vi "Zero_Instruments.vi"(3 "Mode":T5, 5 "Traverse line In":T2 {"Carrier_2 Q (l/min)" format="%#.2f"; "Row Duration (mins)" format="%#.1f"; "Row No" min=0; "Trace Gas Concentration (%)" min=0.0 format="%#_4f"; "Carrier_1 Q (l/min)" format="%#.2f"; "Tunnel Speed" format="%#.2f"; "Start X" format="%#.2f"; "Start Y" format="%#.2f"; "Start Z" format="%#.2f"; "End X" format="%#.2f"; "End Y" format="%#.2f"; "End Z" format="%#.2f"; "Averaging time (min)" min=0.0 format="%#.2f"}) -> (0 "Error Message":string, 1 "Status":T1, 2 "Traverse line Out":T2 {"Carrier_2 Q (l/min)" format="%#.2f"; "Row Duration (mins)" format="%#.1f"; "Row No" min=0; "Trace Gas Concentration (%)" min=0.0 format="%#_4f"; "Carrier_1 Q (l/min)" format="%#.2f"; "Tunnel Speed" format="%#.2f"; "Start X" format="%#.2f"; "Start Y" format="%#.2f"; "Start Z" format="%#.2f"; "End X" format="%#.2f"; "End Y" format="%#.2f"; "End Z" format="%#.2f"; "Averaging time (min)" min=0.0 format="%#.2f"})   [LabVIEW 2017]
uses:
  Gen Trav/Traverse_cluster.ctl
  Gen Trav/Spacing.ctl
  Controls/Multi_run_mode.ctl
  Controls/User_Specific_mode.ctl
  Gen Trav/Multi_Run_Status.ctl
  Controls/Setup.ctl
  Controls/Save_Data.ctl
  Camera Server/Camera enum/Camera resolution.ctl
  Globals/Meas_global.vi
  <vilib>/Analysis/NI_AALPro.lvlib
  <vilib>/Analysis/NI_AALBase.lvlib
panel:
  # "X           Y            Z"
  # "Start"
  # "End"
  # "X           Y            Z"
  # "Start"
  # "End"
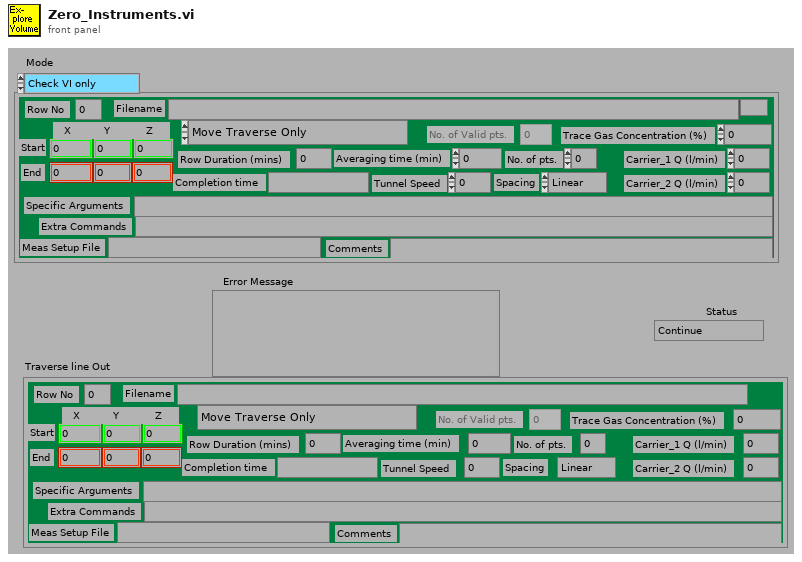
[diagram p1: front panel]
types:
  T1 = typedef "Multi_Run_Status.ctl" = enum16{"Continue", "Continue with Error", "Jump to Next Point", "Jump to Next Row", "Jump To Fall Back", "Terminate Run"}
  T2 = typedef "Traverse_cluster.ctl" = cluster{"Start X":sgl, "Start Y":sgl, "Start Z":sgl, "End X":sgl, "End Y":sgl, "End Z":sgl, "No. of pts.":i32, "Spacing":T3, "Filename":path, "Tunnel Speed":dbl, "Averaging time (min)":dbl, "Extra Commands":string, "Carrier_1 Q (l/min)":dbl, "Carrier_2 Q (l/min)":dbl, "Trace Gas Concentration (%)":dbl, "Specific Arguments":string, "Comments":string, "Row No":i32, "Row Type Selector":T4, "Completion time":string, "Row Duration (mins)":dbl, "No. of Valid pts.":i32, "Meas Setup File":string}
  T3 = typedef "Spacing.ctl" = enum16{"Linear", "Log", "Gauss", "Specified", "N/A"}
  T4 = typedef "Multi_run_mode.ctl" = enum16{"Move Traverse Only", "Set Tunnel Speed Only", "Set Source Only", "Set Measurement Conditions", "Single Measurement", "Vertical Profile", "Lateral Profile", "Longitudinal Profile", "Explore Volume", "Multi-Axis Profile", "Auto Calibrate", "Meas Fast FID Bkgnd", "Check Beam Power", "Scanning Valve Measurement", "Run VI Named:", "Set ADAM Ch", "Wait (minutes)", "Send Message", "Synchronize With:", "Fall Back to this Row", "Turn Off Row Repeating", "Blank Row", "Traverse 3D Volume"}
  T5 = typedef "User_Specific_mode.ctl" = enum16{"Check VI only", "Run VI"}
  T6 = typedef "Save_Data.ctl" = enum16{"Save No Data", "Save Data"}
  T7 = typedef "Setup.ctl" = enum16{"Run Program", "Show Setup", "Save Current Setup", "Setup Front Panel"}
  T8 = typedef "Analysis_info_cluster.ctl" = cluster{"Colour":u32, "Inst type":T9, "Inst name":string, "Symbol":string, "Code name":string, "Extra Info":string, "Inst Array":T10, "Extra Titles":string[], "Extra Values":string[], "U":dbl, "u^2":dbl, "u^3":dbl, "u^4":dbl, "Skew_u":dbl, "Kurt_u":dbl, "Sd Error in Mean":dbl, "% u'/U":dbl, "X":dbl, "Y":dbl, "Z":dbl, "Timescale integral Estimate":dbl, "Sd Error in Variance":dbl, "Calib File":path, "Calib Constants":dbl[], "Output Position":bool, "Full Stats":bool, "Av Sampling Rate":dbl, "Av No of Samples":dbl, "Total Meas Time (s)":dbl, "ADAM Ch Name":string, "Max value":dbl, "Min value":dbl, "Sync Delay Time (s)":dbl}
  T9 = typedef "Inst_type.ctl" = enum16{"Propeller anemometer", "Raw voltage", "Pressure Transducer", "Pitot-static tube", "Preston tube", "Hot wire", "Cross wire 1", "Cross wire 2", "Generic Linear", "Generic Polynomial", "Generic BackPoly", "Fast FID", "Thermocouple", "Cold wire", "Pulsed Wire", "LDA Vel", "LDA Tran time", "LDA Arr time", "Microphone"}
  T10 = typedef "Instrument_Array.ctl" = enum16{"PWA", "LDA", "Analogue"}
  T11 = typedef "Time_Trace_Cluster.ctl" = cluster{"Weighting":dbl[], "Time (s)":dbl[], "Voltage":dbl[], "Eng Values":dbl[]}
  T12 = typedef "Camera resolution.ctl" = u8
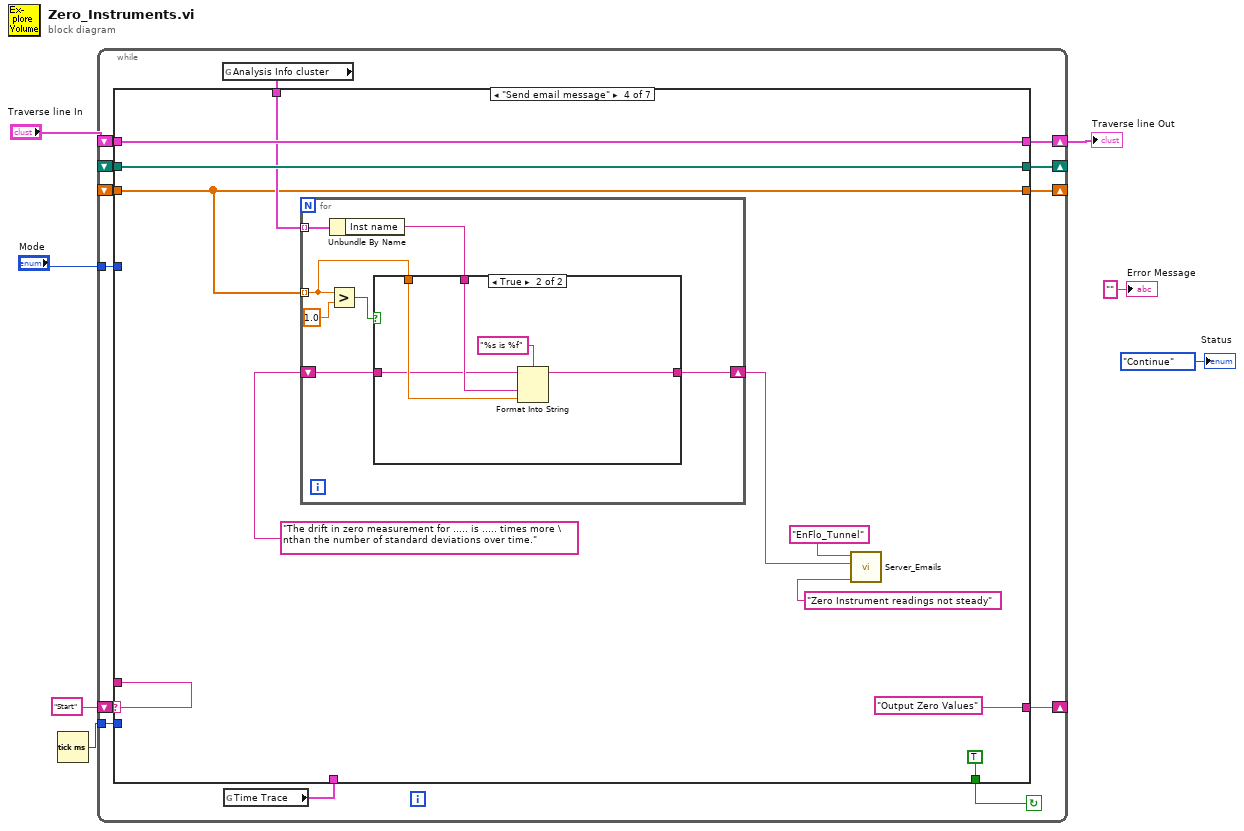
[diagram p0: block diagram]
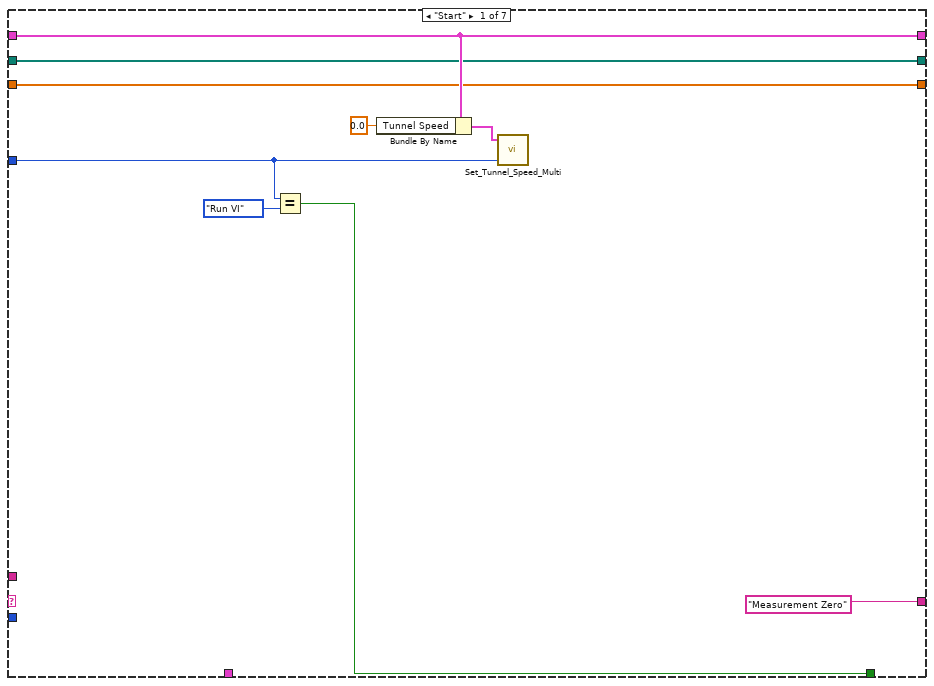
[diagram p2: hidden frame]
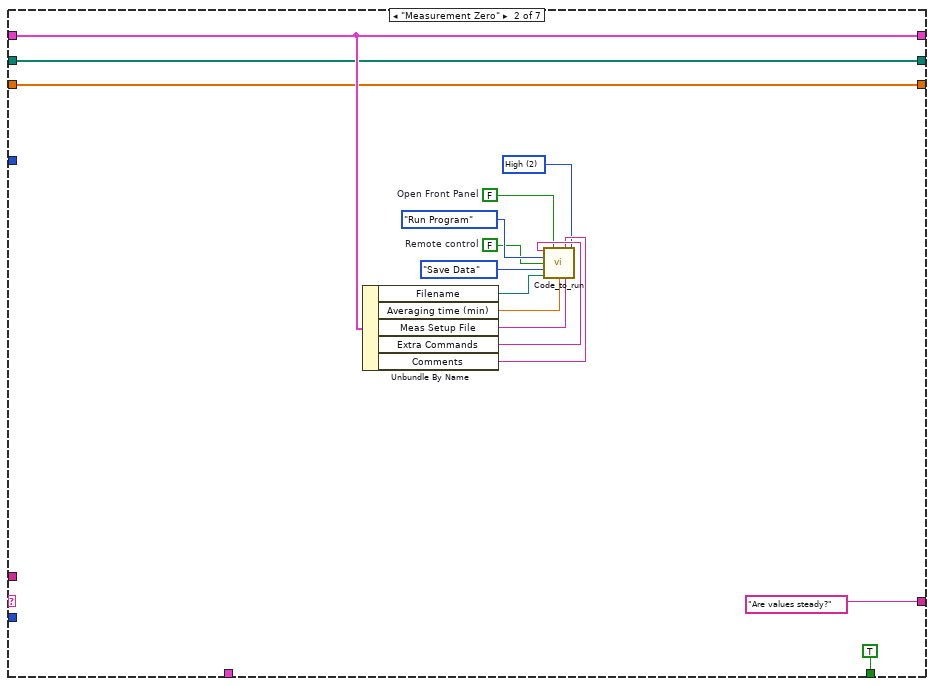
[diagram p3: hidden frame]
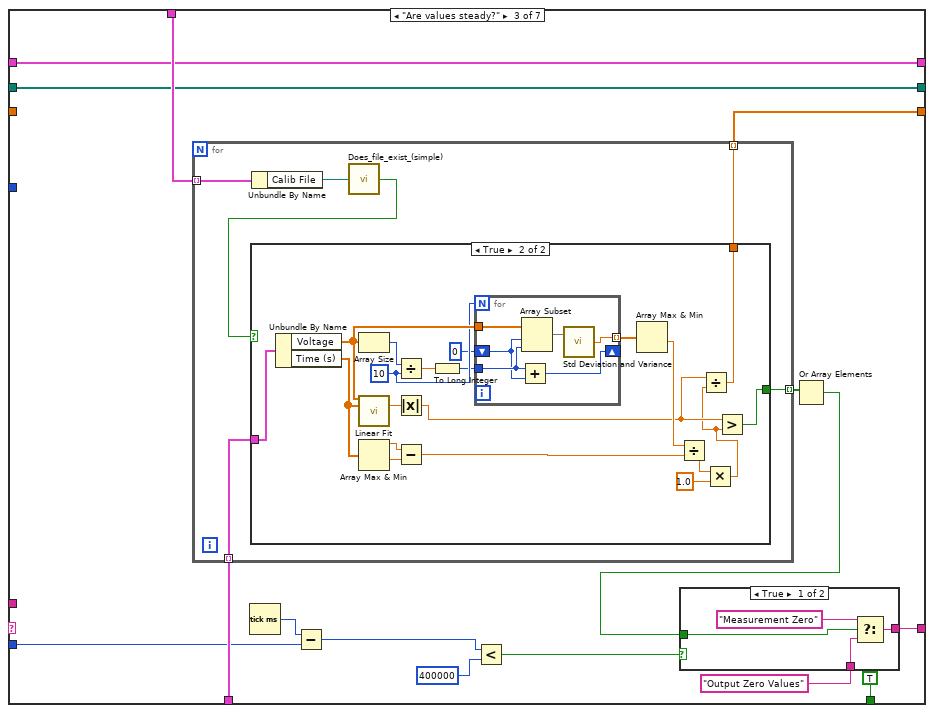
[diagram p4: hidden frame]
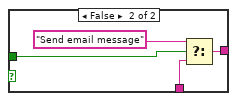
[diagram p5: hidden frame]
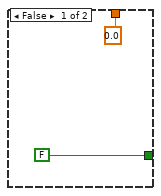
[diagram p6: hidden frame]
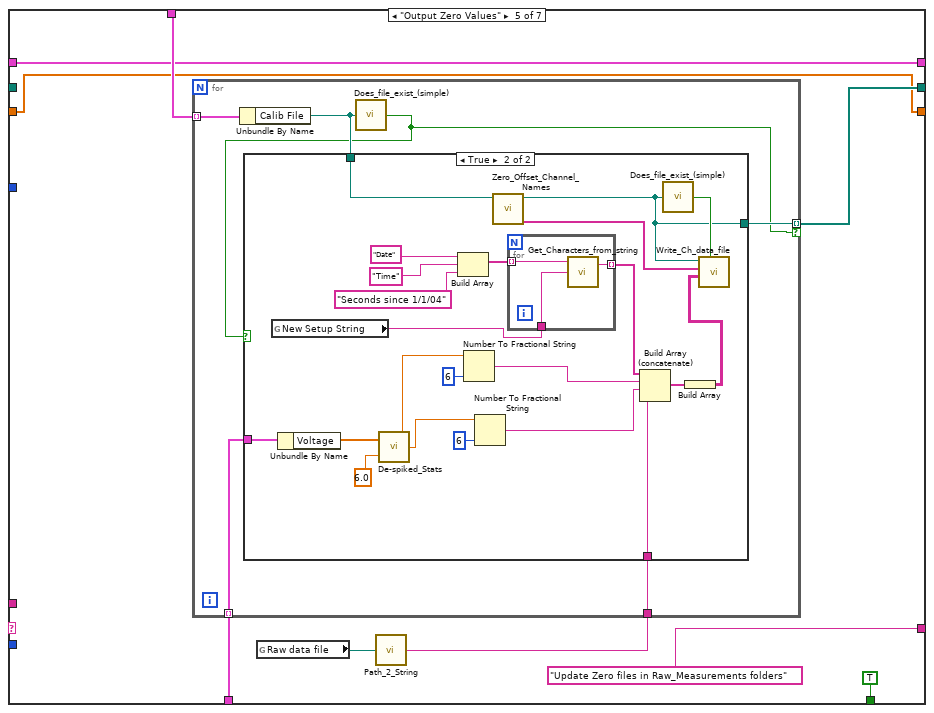
[diagram p8: hidden frame]
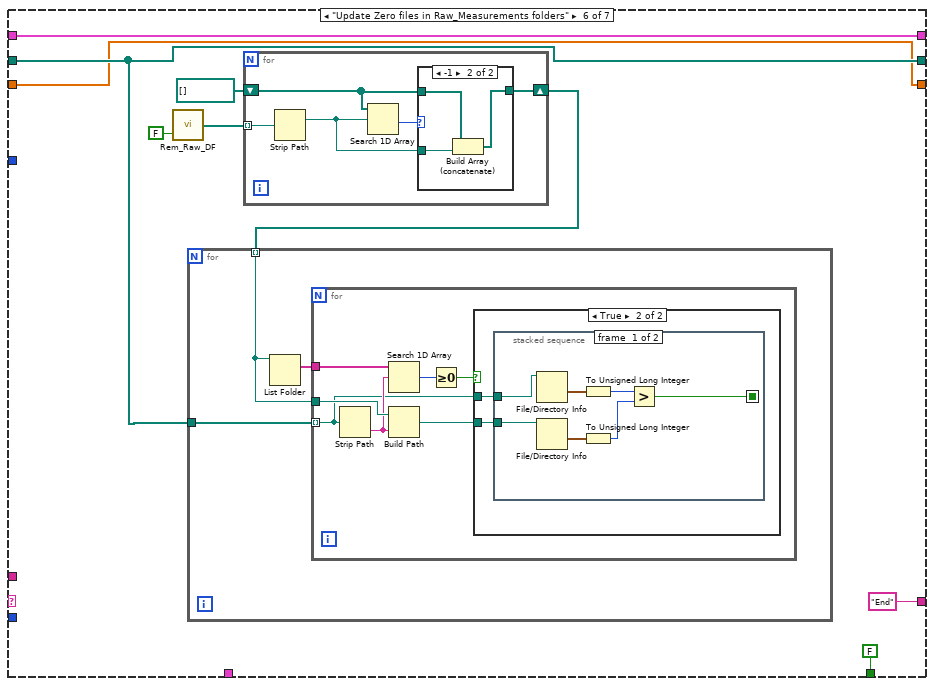
[diagram p10: hidden frame]
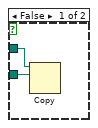
[diagram p11: hidden frame]
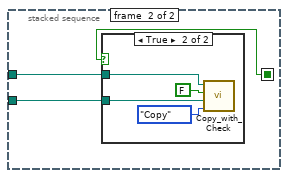
[diagram p12: hidden frame]
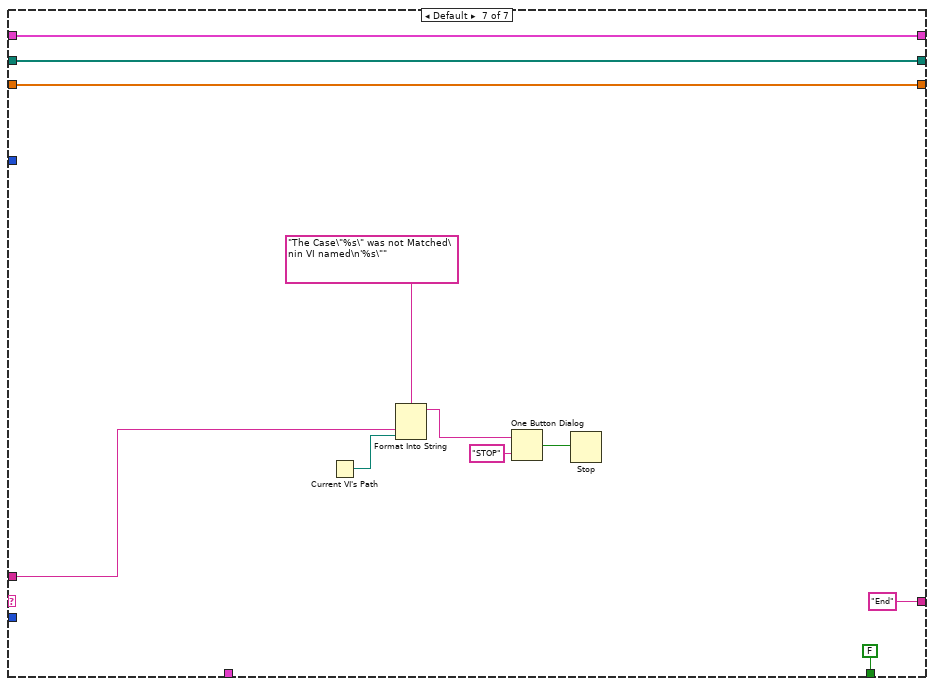
[diagram p15: hidden frame]
diagram:
  n1 = Tick Count (ms)() -> (millisecond timer value=w1:u32)
  n2 = while {
    shift-right: [w16] -> _
    shift-left: "Start" -> [w15]
    shift-right: [w17] -> w5
    shift-left: "Traverse line In" -> [w19]
    tunnel: "Mode" -> [w18]
    tunnel: w1 -> [w12]
    shift-right: [w11] -> _
    shift-left: _ -> [w10]
    shift-right: [w9] -> _
    shift-left: _ -> [w8]
    stop <- w20 continue-if-true
    n3 = global read "Meas_global.vi" "Analysis Info cluster"() -> (w13:T8[])
    n4 = global read "Meas_global.vi" "Time Trace"() -> (w14:T11[])
    n5 = case shown="\"Send email message\"" w15 {
      tunnel: [w24 TRUE TRUE TRUE TRUE FALSE FALSE] -> w20
      tunnel: w19 -> [w27 w33 w56 w110 w130 w174 w214]
      tunnel: w18 -> [w26 _ _ _ _ _ _]
      tunnel: [w27 w33 w56 w110 w130 w174 w214] -> w17
      tunnel: ["Measurement Zero" "Are values steady?" w53 "Output Zero Values" "Update Zero files in Raw_Measurements folders" "End" "End"] -> w16
      tunnel: w15 -> [_ _ _ _ _ _ w217]
      tunnel: w14 -> [_ _ w58 _ w132 _ _]
      tunnel: w13 -> [_ _ w57 w108 w131 _ _]
      tunnel: w12 -> [_ _ w51 _ _ _ _]
      tunnel: [w22 w31 w49 w109 w126 w169 w213] -> w11
      tunnel: w10 -> [w22 w31 w49 w109 _ w169 w213]
      tunnel: [w21 w30 w45 w102 w125 w166 w212] -> w9
      tunnel: w8 -> [w21 w30 _ w102 w125 w166 w212]
      frame "Start" {
        n6 = Equal?(x=w26, y=User_Specific_mode."Run VI") -> (x = y?=w24:bool)
        n7 = Bundle By Name(cluster=w27, "Tunnel Speed"=0.0) -> (w29:T2)
        n8 = call "Set_Tunnel_Speed_Multi.vi"("Simulate/Run"=w26, "Traverse line"=w29) -> ()  [unwired: 4 out]
      }
      frame "Measurement Zero" {
        w37 = T12 2 items=["Low", "Med.", "High", "Max."] ("Camera Resolution")
        w38 = FALSE  # Open Front Panel
        w35 = FALSE  # Remote control
        n9 = Unbundle By Name(w33) -> ("Filename"=w43:path, "Averaging time (min)"=w42:dbl, "Meas Setup File"=w41:string, "Extra Commands"=w40:string, "Comments"=w39:string)
        n10 = call "Code_to_run.vi"("Extra command String"=w40, "Open Front Panel"=w38, "Current Row Comments"=w39, "Camera Resolution"=w37, "setup"=Setup."Run Program", "Remote control"=w35, "File"=Save_Data."Save Data", "Results Filename"=w43, "Averaging time (min)"=w42, "Setup filename"=w41) -> ()  [unwired: 2 in, 4 out]
      }
      frame "Are values steady?" {
        n11 = for {
          tunnel: w57 -> [w73] mode=indexing
          tunnel: w58 -> [w70] mode=indexing
          tunnel: [w69] -> w55 mode=indexing
          tunnel: [w68] -> w45 mode=indexing
          n12 = Unbundle By Name(w73) -> ("Calib File"=w72:path)
          n13 = call "Does_file_exist_(simple).vi"("Pathname"=w72) -> ("exists?"=w71:bool)
          n14 = case shown="True" w71 {
            tunnel: w70 -> [_ w82]
            tunnel: [FALSE w80] -> w69
            tunnel: [0.0 w76] -> w68
            frame False {
            }
            frame True {
              w88 = 10 ("y")
              n15 = Unbundle By Name(w82) -> ("Voltage"=w95:dbl[], "Time (s)"=w90:dbl[])
              n16 = Array Size(array=w95) -> (size(s)=w84:i32)
              n17 = call <vilib>:"Linear Fit.vi"("Y"=w95, "X"=w90) -> ("slope"=w83:dbl)  [unwired: 9 in, 4 out]
              n18 = Array Max & Min(array=w90) -> (max value=w91:dbl, min value=w92:dbl)  [unwired: 2 out]
              n19 = Divide(x=w84, y=w88) -> (x/y=w86:dbl)
              n20 = Absolute Value(x=w83) -> (abs(x)=w78:dbl)
              n21 = Subtract(x=w91, y=w92) -> (x-y=w94:dbl)
              n22 = To Long Integer(number=w86) -> (32bit integer=w87:i32)
              n23 = for {
                N: w88 -> [_]
                tunnel: w95 -> [w101]
                shift-right: [w98] -> _
                shift-left: 0 ("y") -> [w99]
                tunnel: w87 -> [w100]
                tunnel: [w96] -> w89 mode=indexing
                n24 = Add(x=w100, y=w99) -> (x+y=w98:i32)
                n25 = Array Subset(array=w101, index=w99, length=w100) -> (w97:dbl[])
                n26 = call <vilib>:"Std Deviation and Variance.vi"("X"=w97) -> ("standard deviation"=w96:dbl)  [unwired: 1 in, 2 out]
              }
              n27 = Array Max & Min(array=w89) -> (min value=w93:dbl)  [unwired: 3 out]
              n28 = Divide(x=w93, y=w94) -> (x/y=w81:dbl)
              n29 = Multiply(x=w81, y=1.0) -> (x*y=w77:dbl)
              n30 = Divide(x=w78, y=w77) -> (x/y=w76:dbl)
              n31 = Greater?(x=w78, y=w77) -> (0:w80:bool)
            }
          }
        }
        n32 = Tick Count (ms)() -> (millisecond timer value=w52:u32)
        n33 = Subtract(x=w52, y=w51) -> (x-y=w50:u32)
        n34 = Less?(x=w50, y=u32 400000) -> (x < y?=w48:bool)
        n35 = Or Array Elements(Boolean array=w55) -> (logical OR=w47:bool)
        n36 = case shown="True" w48 {
          tunnel: [w63 w67] -> w53
          tunnel: w47 -> [w61 w66]
          tunnel: "Output Zero Values" -> [w60 w64]
          frame True {
            n37 = Select(t="Measurement Zero", s=w61, f=w60) -> (s? t:f=w63:string)
          }
          frame False {
            n38 = Select(t="Send email message", s=w66, f=w64) -> (s? t:f=w67:string)
          }
        }
      }
      frame "Send email message" {
        n39 = for {
          tunnel: w108 -> [w118] mode=indexing
          tunnel: w102 -> [w114] mode=indexing
          shift-right: [w112] -> w103
          shift-left: "The drift in zero measurement for ..... is ..... times more \nthan the number of standard deviations over time." -> [w113]
          n40 = Greater?(x=w114, y=1.0) -> (0:w116:bool)
          n41 = Unbundle By Name(w118) -> ("Inst name"=w115:string)
          n42 = case shown="True" w116 {
            tunnel: w115 -> [_ w124]
            tunnel: w114 -> [_ w123]
            tunnel: w113 -> [w119 w122]
            tunnel: [w119 w121] -> w112
            frame False {
            }
            frame True {
              n43 = Format Into String(format string="%s is %f", initial string=w122, w124, w123) -> (resulting string=w121:string)  [unwired: 1 in, 1 out]
            }
          }
        }
        n44 = call "Server_Emails.vi"("Client Name Contains"="EnFlo_Tunnel", "Message"=w103, "Subject"="Zero Instrument readings not steady" ("Error Type")) -> ()  [unwired: 2 in, 3 out]
      }
      frame "Output Zero Values" {
        n45 = global read "Meas_global.vi" "Raw data file"() -> (w128:path)
        n46 = call "Path_2_String.vi"("Real Path"=w128) -> ("Path String"=w127:string)
        n47 = for {
          tunnel: w131 -> [w139] mode=indexing
          tunnel: w132 -> [w138] mode=indexing
          tunnel: w127 -> [w137]
          tunnel: [w135] -> w126 mode=indexing if=w134
          n48 = Unbundle By Name(w139) -> ("Calib File"=w136:path)
          n49 = call "Does_file_exist_(simple).vi"("Pathname"=w136) -> ("exists?"=w134:bool)
          n50 = case shown="True" w134 {
            tunnel: w138 -> [_ w162]
            tunnel: w137 -> [_ w146]
            tunnel: w136 -> [w140 w142]
            tunnel: [w140 w141] -> w135
            frame False {
            }
            frame True {
              n51 = global read "Meas_global.vi" "New Setup String"() -> (w150:string)
              n52 = Unbundle By Name(w162) -> ("Voltage"=w160:dbl[])
              n53 = call "De-spiked_Stats.vi"("Raw Signal"=w160, "No of st dev to chop at"=6.0) -> ("mean"=w156:dbl, "standard deviation"=w157:dbl)  [unwired: 1 out]
              n54 = Build Array("Date", "Time", "Seconds since 1/1/04") -> (w151:string[])
              n55 = Number To Fractional String(number=w156, precision (6)=i16 6) -> (F-format string=w148:string)  [unwired: 2 out]
              n56 = Number To Fractional String(number=w157, precision (6)=i16 6) -> (F-format string=w147:string)  [unwired: 2 out]
              n57 = call "Zero_Offset_Channel_Names.vi"("Calib Filename"=w142) -> ("Channel names"=w145:string[], "Zero Filename"=w141:path)  [unwired: 3 in, 2 out]
              n58 = for {
                tunnel: w151 -> [w165] mode=indexing
                tunnel: w150 -> [w164]
                tunnel: [w163] -> w149 mode=indexing
                n59 = call "Get_Characters_from_string.vi"("Input string"=w164, "Variable name"=w165) -> ("Value"=w163:string)  [unwired: 1 in, 1 out]
              }
              n60 = Build Array (concatenate)(w149, w148, w147, w146) -> (w144:string[])
              n61 = call "Does_file_exist_(simple).vi"("Pathname"=w141) -> ("exists?"=w155:bool)
              n62 = Build Array(w144) -> (w143:string[][])
              n63 = call "Write_Ch_data_file.vi"("exists?"=w155, "Channel Values"=w143, "Channel names"=w145, "Filename"=w141) -> ()  [unwired: 4 in, 4 out]
            }
          }
        }
      }
      frame "Update Zero files in Raw_Measurements folders" {
        n64 = call "Rem_Raw_DF.vi"("Clear History?"=FALSE) -> ("List of Filenames"=w172:path[])  [unwired: 1 in]
        n65 = for {
          tunnel: w172 -> [w207] mode=indexing
          shift-right: [w203] -> w170
          shift-left: path[] [] -> [w205]
          n66 = Strip Path(path=w207) -> (stripped path=w204:path)  [unwired: 1 out]
          n67 = Search 1D Array(1D array=w205, element=w204) -> (index of element=w206:i32)  [unwired: 1 in]
          n68 = case shown="-1" w206 {
            tunnel: w205 -> [w208 w211]
            tunnel: w204 -> [_ w210]
            tunnel: [w208 w209] -> w203
            frame Default {
            }
            frame -1 {
              n69 = Build Array (concatenate)(w211, w210) -> (w209:path[])
            }
          }
        }
        n70 = for {
          tunnel: w170 -> [w176] mode=indexing
          tunnel: w169 -> [w175]
          n71 = List Folder(path=w176) -> (filenames=w177:string[])  [unwired: 1 in, 5 out]
          n72 = for {
            tunnel: w175 -> [w178] mode=indexing
            tunnel: w176 -> [w181]
            tunnel: w177 -> [w184]
            n73 = Strip Path(path=w178) -> (name=w180:string)  [unwired: 1 out]
            n74 = Search 1D Array(1D array=w184, element=w180) -> (index of element=w183:i32)  [unwired: 1 out]
            n75 = Build Path(base path=w181, name or relative path=w180) -> (appended path=w179:path)
            n76 = Greater Or Equal To 0?(x=w183) -> (x >= 0?=w182:bool)
            n77 = case shown="True" w182 {
              tunnel: w179 -> [w186 w187]
              tunnel: w178 -> [w185 w188]
              frame False {
                n78 = Copy(10:w186, 11:w185) -> ()  [unwired: 1 in, 5 out]
              }
              frame True {
                n79 = stacked-sequence {
                  seq-local: [w191 _] -> [_ w198]
                  tunnel: w188 -> [w195 w196]
                  tunnel: w187 -> [w194 w197]
                  frame #0 {
                    n80 = File/Directory Info(path=w195) -> (last mod=w189:timestamp)  [unwired: 1 in, 6 out]
                    n81 = File/Directory Info(path=w194) -> (last mod=w190:timestamp)  [unwired: 1 in, 6 out]
                    n82 = To Unsigned Long Integer(number=w189) -> (unsigned 32bit integer=w193:u32)
                    n83 = To Unsigned Long Integer(number=w190) -> (unsigned 32bit integer=w192:u32)
                    n84 = Greater?(x=w193, y=w192) -> (0:w191:bool)
                  }
                  frame #1 {
                    n85 = case shown="True" w198 {
                      tunnel: w197 -> [_ w201]
                      tunnel: w196 -> [_ w202]
                      frame False {
                      }
                      frame True {
                        n86 = call "Copy_with_Check.vi"("Mode"=enum16{"Move", "Copy"}."Copy", "Target Path"=w201, "Variable Target?"=FALSE, "Source Path"=w202) -> ()  [unwired: 1 out]
                      }
                    }
                  }
                }
              }
            }
          }
        }
      }
      frame Default {
        n87 = Current VI's Path() -> (path=w222:path)
        n88 = Format Into String(format string="The Case\"%s\" was not Matched\nin VI named\n'%s\"" ("Format String"), w217, w222) -> (resulting string=w219:string)  [unwired: 2 in, 1 out]
        n89 = One Button Dialog(message=w219, button name ("OK")="STOP") -> (true=w221:bool)
        n90 = Stop(stop? (T)=w221) -> ()
      }
    }
  }
  "Traverse line Out" <- w5
  "Error Message" <- "" ("Error Message")
  "Status" <- Multi_Run_Status."Continue" ("Status")
